vi "begin_DriveQuadTalonSrxl.vi"(0 "Time":T1, 3 "Gear Ratio":dbl=1.0 format="%.4f", 4 "Distance Type":T2, 5 "Enc Edges / Rev":dbl=1440.0 format="%.4f", 6 "Wheel Radius In":dbl=3.0 format="%.4f", 7 "MAX DESIRED\nVELOCITY\n(UNITS)":dbl=5800.0 format="%#_13g", 8 "Right Slave CAN":u8=12, 9 "RIght Master CAN":u8=10, 10 "Left Slave CAN":u8=13, 11 "Left Master CAN":u8=14) -> ()   [LabVIEW 2019, in "DriveQuadTalonSRX_Motor.lvlib"]
doc: "Open drives for 4 motor arcade drive using Talon SRX controllers. Configure for velocity control using directly wired encoders on master talon."
uses:
  DriveQuadTalonSRX_Motor.lvlib
  Dist_Type.ctl
  Time_Units_Control.ctl
  <vilib>/Rock Robotics/WPI/SafetyOutput/WPI_SafetyOutputConfigMenu.ctl
  <vilib>/Rock Robotics/WPI/ThirdParty/Phoenix-LabVIEW/Motor Controller/Controls/CTRE_Phoenix_MotorControl_FeedbackDevice.ctl
  <vilib>/Rock Robotics/WPI/ThirdParty/Phoenix-LabVIEW/Motor Controller/Controls/CTRE_Phoenix_MotorControl_NeutralMode.ctl
  globals_DriveQuadTalonSRX.vi
  <vilib>/Rock Robotics/WPI/RobotDrive/WPI_RobotDriveOpen2MotorWithExistingMotors.vi
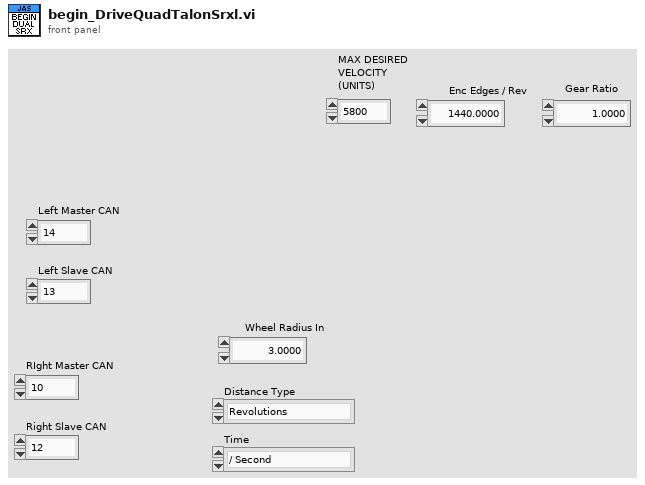
[diagram p1: front panel]
types:
  T1 = typedef "DriveQuadTalonSRX_Motor.lvlib/Time_Units_Control.ctl" = enum16{"/ Second", "/ Minute"}
  T2 = typedef "DriveQuadTalonSRX_Motor.lvlib/Dist_Type.ctl" = enum16{"Revolutions", "Feet"}
  T3 = typedef "CTRE_Phoenix_MotorControl_NeutralMode.ctl" = enum8{"EEPROMSetting", "Override to Coast", "Override to Brake"}
  T4 = typedef "WPI_SafetyOutputConfigMenu.ctl" = enum16{"Enable", "Disable"}
  T5 = enum16{"FollowerType_PercentOutput", "FollowerType_AuxOutput1"}
  T6 = typedef "CTRE_Phoenix_MotorControl_FeedbackDevice.ctl" = i8
  T7 = typedef "WPI_MotorControlDeviceRef.ctl" = cluster{"DeviceStatus":errorcluster, "Type":T8, "PWM":cluster{"PWM Channel":T9, "DeadBand":T10}, "CAN":cluster{"Device Number":u8, "SetOutput VI Ref":variant, "GetOutput VI Ref":variant, "Enable VI Ref":variant, "Disable VI Ref":variant, "Data":variant}, "Invert":bool, "DIO PWM":cluster{"PWM \"Enable\" Channel":T9, "DIOChannel":T11, "PWM Rate":dbl}}
  T8 = typedef "WPI_MotorControlType.ctl" = enum16{"PWM", "CAN", "DIO PWM"}
  T9 = typedef "FPGA_DIOPWMChannel.ctl" = enum8{"PWM 0", "PWM 1", "PWM 2", "PWM 3", "PWM 4", "PWM 5", "PWM 6", "PWM 7", "PWM 8", "PWM 9", "PWM MXP 0", "PWM MXP 1", "PWM MXP 2", "PWM MXP 3", "PWM MXP 4", "PWM MXP 5", "PWM MXP 6", "PWM MXP 7", "PWM MXP 8", "PWM MXP 9", "Invalid"}
  T10 = typedef "WPI_PWMDeadband.ctl" = cluster{"Name":string, "maxPositivePwm":i32, "minPositivePwm":i32, "centerPwm":i32, "maxNegativePwm":i32, "minNegativePwm":i32, "angularRange":u16}
  T11 = typedef "FPGA_DIOChannel.ctl" = enum8{"DIO 0", "DIO 1", "DIO 2", "DIO 3", "DIO 4", "DIO 5", "DIO 6", "DIO 7", "DIO 8", "DIO 9", "DIO MXP 0", "DIO MXP 1", "DIO MXP 2", "DIO MXP 3", "DIO MXP 4", "DIO MXP 5", "DIO MXP 6", "DIO MXP 7", "DIO MXP 8", "DIO MXP 9", "DIO MXP 10", "DIO MXP 11", "DIO MXP 12", "DIO MXP 13", "DIO MXP 14", "DIO MXP 15", "SPI Port CS1", "SPI Port CS2", "SPI Port CS3", "SPI Port MISO", "SPI Port MOSI", "Invalid"}
  T12 = typedef "WPI_RobotDriveDevRef.ctl" = cluster{"DevStatus":errorcluster, "Motors[]":T7[], "Square Inputs":bool, "Max Output":dbl}
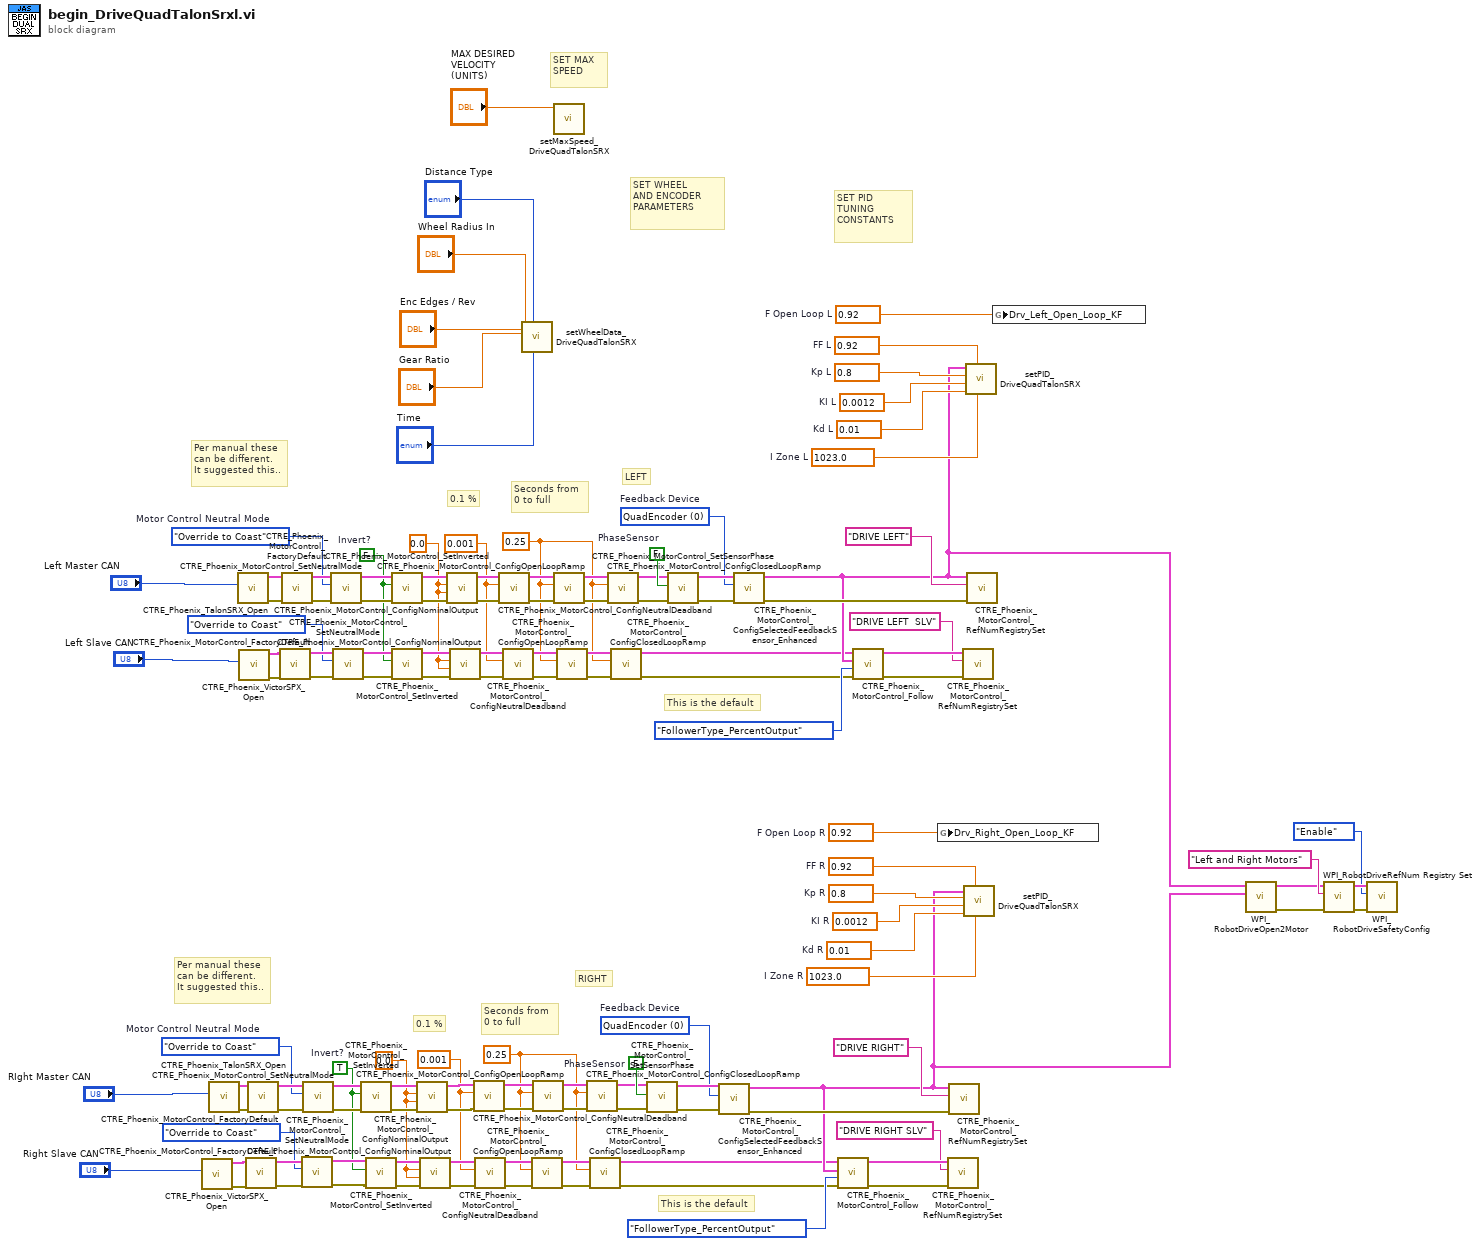
[diagram p0: block diagram]
diagram:
  w4 = 0.25 ("secondsFromNeutralToFull")
  w5 = 0.001 ("Percent Deadband")
  w6 = 0.0 ("Forward Nominal Percent Output")
  w27 = 0.25 ("secondsFromNeutralToFull")
  w28 = 0.001 ("Percent Deadband")
  w29 = 0.0 ("Forward Nominal Percent Output")
  w91 = 0.92  # F Open Loop L
  w97 = 1023.0  # I Zone L
  w98 = 0.01  # Kd L
  w99 = 0.0012  # KI L
  w100 = 0.8  # Kp L
  w101 = 0.92  # FF L
  w92 = 1023.0  # I Zone R
  w93 = 0.01  # Kd R
  w94 = 0.0012  # KI R
  w95 = 0.8  # Kp R
  w96 = 0.92  # FF R
  w90 = 0.92  # F Open Loop R
  w77 = FALSE  # Invert?
  w66 = TRUE  # Invert?
  w116 = T6 0 items=["None"=-1, "QuadEncoder"=0, "Analog"=2, "Tachometer"=4, "Pulse Width Encoded Position"=8, "Sensor Sum (S0 + S1)"=9, "Sensor Difference (D0 - D1)"=10, "Remote Source 0"=11, "Remote Source 1"=12, "Software Emulated"=15]  # Feedback Device
  w115 = T6 0 items=["None"=-1, "QuadEncoder"=0, "Analog"=2, "Tachometer"=4, "Pulse Width Encoded Position"=8, "Sensor Sum (S0 + S1)"=9, "Sensor Difference (D0 - D1)"=10, "Remote Source 0"=11, "Remote Source 1"=12, "Software Emulated"=15]  # Feedback Device
  w64 = CTRE_Phoenix_MotorControl_NeutralMode."Override to Coast"  # Motor Control Neutral Mode
  w76 = CTRE_Phoenix_MotorControl_NeutralMode."Override to Coast"  # Motor Control Neutral Mode
  w65 = FALSE  # PhaseSensor
  w104 = FALSE  # PhaseSensor
  # "This is the default"
  # "This is the default"
  # "Per manual these\ncan be different.  \nIt suggested this.."
  # "Per manual these\ncan be different.  \nIt suggested this.."
  # "Seconds from\n0 to full"
  # "Seconds from\n0 to full"
  # "0.1 %"
  # "0.1 %"
  # "SET PID\nTUNING\nCONSTANTS"
  # "SET WHEEL\nAND ENCODER\nPARAMETERS"
  # "SET MAX\nSPEED"
  # "RIGHT"
  # "LEFT"
  n1 = call <vilib>:"CTRE_Phoenix_VictorSPX_Open.vi"("Device Number"="Right Slave CAN") -> ("error out"=w63:errorcluster, "CAN Talon SRX Ref"=w62:T7)  [unwired: 9 in]
  n2 = call <vilib>:"CTRE_Phoenix_TalonSRX_Open.vi"("Device Number"="RIght Master CAN") -> ("error out"=w110:errorcluster, "CAN Talon SRX Ref"=w109:T7)  [unwired: 9 in]
  n3 = call <vilib>:"CTRE_Phoenix_TalonSRX_Open.vi"("Device Number"="Left Master CAN") -> ("error out"=w106:errorcluster, "CAN Talon SRX Ref"=w105:T7)  [unwired: 9 in]
  n4 = call <vilib>:"CTRE_Phoenix_VictorSPX_Open.vi"("Device Number"="Left Slave CAN") -> ("error out"=w60:errorcluster, "CAN Talon SRX Ref"=w59:T7)  [unwired: 9 in]
  n5 = call <vilib>:"CTRE_Phoenix_MotorControl_FactoryDefault.vi"("error in"=w63, "PhoenixMotorControlDevRef"=w62) -> ("error out"=w69:errorcluster, "PhoenixMotorControlDevRef"=w70:T7)  [unwired: 8 in]
  n6 = call <vilib>:"CTRE_Phoenix_MotorControl_FactoryDefault.vi"("error in"=w110, "PhoenixMotorControlDevRef"=w109) -> ("error out"=w114:errorcluster, "PhoenixMotorControlDevRef"=w113:T7)  [unwired: 8 in]
  n7 = call <vilib>:"CTRE_Phoenix_MotorControl_FactoryDefault.vi"("error in"=w60, "PhoenixMotorControlDevRef"=w59) -> ("error out"=w81:errorcluster, "PhoenixMotorControlDevRef"=w80:T7)  [unwired: 8 in]
  n8 = call <vilib>:"CTRE_Phoenix_MotorControl_FactoryDefault.vi"("error in"=w106, "PhoenixMotorControlDevRef"=w105) -> ("error out"=w112:errorcluster, "PhoenixMotorControlDevRef"=w111:T7)  [unwired: 8 in]
  n9 = call <vilib>:"CTRE_Phoenix_MotorControl_SetNeutralMode.vi"("error in (no error)"=w69, "Motor Control Neutral Mode"=CTRE_Phoenix_MotorControl_NeutralMode."Override to Coast", "PhoenixMotorControlDevRef"=w70) -> ("error out"=w75:errorcluster, "PhoenixMotorControlDevRef"=w74:T7)  [unwired: 7 in]
  n10 = call <vilib>:"CTRE_Phoenix_MotorControl_SetNeutralMode.vi"("error in (no error)"=w114, "Motor Control Neutral Mode"=w64, "PhoenixMotorControlDevRef"=w113) -> ("error out"=w121:errorcluster, "PhoenixMotorControlDevRef"=w122:T7)  [unwired: 7 in]
  n11 = call <vilib>:"CTRE_Phoenix_MotorControl_SetNeutralMode.vi"("error in (no error)"=w112, "Motor Control Neutral Mode"=w76, "PhoenixMotorControlDevRef"=w111) -> ("error out"=w118:errorcluster, "PhoenixMotorControlDevRef"=w117:T7)  [unwired: 7 in]
  n12 = call <vilib>:"CTRE_Phoenix_MotorControl_SetNeutralMode.vi"("error in (no error)"=w81, "Motor Control Neutral Mode"=CTRE_Phoenix_MotorControl_NeutralMode."Override to Coast", "PhoenixMotorControlDevRef"=w80) -> ("error out"=w78:errorcluster, "PhoenixMotorControlDevRef"=w79:T7)  [unwired: 7 in]
  n13 = call <vilib>:"CTRE_Phoenix_MotorControl_SetInverted.vi"("error in (no error)"=w121, "Invert?"=w66, "PhoenixMotorControlDevRef"=w122) -> ("error out"=w16:errorcluster, "PhoenixMotorControlDevRef"=w26:T7)  [unwired: 7 in]
  n14 = call <vilib>:"CTRE_Phoenix_MotorControl_SetInverted.vi"("error in (no error)"=w75, "Invert?"=w66, "PhoenixMotorControlDevRef"=w74) -> ("error out"=w11:errorcluster, "PhoenixMotorControlDevRef"=w21:T7)  [unwired: 7 in]
  n15 = call <vilib>:"CTRE_Phoenix_MotorControl_SetInverted.vi"("error in (no error)"=w118, "Invert?"=w77, "PhoenixMotorControlDevRef"=w117) -> ("error out"=w48:errorcluster, "PhoenixMotorControlDevRef"=w49:T7)  [unwired: 7 in]
  n16 = call <vilib>:"CTRE_Phoenix_MotorControl_SetInverted.vi"("error in (no error)"=w78, "Invert?"=w77, "PhoenixMotorControlDevRef"=w79) -> ("error out"=w36:errorcluster, "PhoenixMotorControlDevRef"=w37:T7)  [unwired: 7 in]
  n17 = call <vilib>:"CTRE_Phoenix_MotorControl_ConfigNominalOutput.vi"("error in (no error)"=w16, "Reverse Nominal Percent Output"=w6, "Forward Nominal Percent Output"=w6, "PhoenixMotorControlDevRef"=w26) -> ("error out"=w15:errorcluster, "PhoenixMotorControlDevRef"=w25:T7)  [unwired: 6 in]
  n18 = call <vilib>:"CTRE_Phoenix_MotorControl_ConfigNominalOutput.vi"("error in (no error)"=w11, "Reverse Nominal Percent Output"=w6, "Forward Nominal Percent Output"=w6, "PhoenixMotorControlDevRef"=w21) -> ("error out"=w10:errorcluster, "PhoenixMotorControlDevRef"=w20:T7)  [unwired: 6 in]
  n19 = call <vilib>:"CTRE_Phoenix_MotorControl_ConfigNominalOutput.vi"("error in (no error)"=w48, "Reverse Nominal Percent Output"=w29, "Forward Nominal Percent Output"=w29, "PhoenixMotorControlDevRef"=w49) -> ("error out"=w46:errorcluster, "PhoenixMotorControlDevRef"=w47:T7)  [unwired: 6 in]
  n20 = call <vilib>:"CTRE_Phoenix_MotorControl_ConfigNominalOutput.vi"("error in (no error)"=w36, "Reverse Nominal Percent Output"=w29, "Forward Nominal Percent Output"=w29, "PhoenixMotorControlDevRef"=w37) -> ("error out"=w32:errorcluster, "PhoenixMotorControlDevRef"=w35:T7)  [unwired: 6 in]
  n21 = call <vilib>:"CTRE_Phoenix_MotorControl_ConfigNeutralDeadband.vi"("error in (no error)"=w15, "Percent Deadband"=w5, "PhoenixMotorControlDevRef"=w25) -> ("error out"=w14:errorcluster, "PhoenixMotorControlDevRef"=w24:T7)  [unwired: 7 in]
  n22 = call <vilib>:"CTRE_Phoenix_MotorControl_ConfigNeutralDeadband.vi"("error in (no error)"=w10, "Percent Deadband"=w5, "PhoenixMotorControlDevRef"=w20) -> ("error out"=w9:errorcluster, "PhoenixMotorControlDevRef"=w19:T7)  [unwired: 7 in]
  n23 = call <vilib>:"CTRE_Phoenix_MotorControl_ConfigNeutralDeadband.vi"("error in (no error)"=w46, "Percent Deadband"=w28, "PhoenixMotorControlDevRef"=w47) -> ("error out"=w44:errorcluster, "PhoenixMotorControlDevRef"=w45:T7)  [unwired: 7 in]
  n24 = call <vilib>:"CTRE_Phoenix_MotorControl_ConfigNeutralDeadband.vi"("error in (no error)"=w32, "Percent Deadband"=w28, "PhoenixMotorControlDevRef"=w35) -> ("error out"=w31:errorcluster, "PhoenixMotorControlDevRef"=w34:T7)  [unwired: 7 in]
  n25 = call "setWheelData_DriveQuadTalonSRX.vi"("Time"="Time", "Distance Type"="Distance Type", "Enc Edges / Rev"="Enc Edges / Rev", "Gear Ratio"="Gear Ratio", "Wheel Radius In"="Wheel Radius In") -> ()  [unwired: 2 in, 5 out]
  n26 = call <vilib>:"CTRE_Phoenix_MotorControl_ConfigOpenLoopRamp.vi"("error in (no error)"=w9, "secondsFromNeutralToFull"=w4, "PhoenixMotorControlDevRef"=w19) -> ("error out"=w8:errorcluster, "PhoenixMotorControlDevRef"=w18:T7)  [unwired: 7 in]
  n27 = call <vilib>:"CTRE_Phoenix_MotorControl_ConfigOpenLoopRamp.vi"("error in (no error)"=w14, "secondsFromNeutralToFull"=w4, "PhoenixMotorControlDevRef"=w24) -> ("error out"=w13:errorcluster, "PhoenixMotorControlDevRef"=w23:T7)  [unwired: 7 in]
  n28 = call "setMaxSpeed_DriveQuadTalonSRX.vi"("MAX DESIRED\nVELOCITY (UNITS)"="MAX DESIRED\nVELOCITY\n(UNITS)") -> ()  [unwired: 8 in, 2 out]
  n29 = call <vilib>:"CTRE_Phoenix_MotorControl_ConfigOpenLoopRamp.vi"("error in (no error)"=w44, "secondsFromNeutralToFull"=w27, "PhoenixMotorControlDevRef"=w45) -> ("error out"=w42:errorcluster, "PhoenixMotorControlDevRef"=w43:T7)  [unwired: 7 in]
  n30 = call <vilib>:"CTRE_Phoenix_MotorControl_ConfigOpenLoopRamp.vi"("error in (no error)"=w31, "secondsFromNeutralToFull"=w27, "PhoenixMotorControlDevRef"=w34) -> ("error out"=w30:errorcluster, "PhoenixMotorControlDevRef"=w33:T7)  [unwired: 7 in]
  n31 = call <vilib>:"CTRE_Phoenix_MotorControl_ConfigClosedLoopRamp.vi"("error in (no error)"=w13, "secondsFromNeutralToFull"=w4, "PhoenixMotorControlDevRef"=w23) -> ("error out"=w12:errorcluster, "PhoenixMotorControlDevRef"=w22:T7)  [unwired: 7 in]
  n32 = call <vilib>:"CTRE_Phoenix_MotorControl_ConfigClosedLoopRamp.vi"("error in (no error)"=w8, "secondsFromNeutralToFull"=w4, "PhoenixMotorControlDevRef"=w18) -> ("error out"=w7:errorcluster, "PhoenixMotorControlDevRef"=w17:T7)  [unwired: 7 in]
  n33 = call <vilib>:"CTRE_Phoenix_MotorControl_ConfigClosedLoopRamp.vi"("error in (no error)"=w42, "secondsFromNeutralToFull"=w27, "PhoenixMotorControlDevRef"=w43) -> ("error out"=w41:errorcluster, "PhoenixMotorControlDevRef"=w40:T7)  [unwired: 7 in]
  n34 = call <vilib>:"CTRE_Phoenix_MotorControl_ConfigClosedLoopRamp.vi"("error in (no error)"=w30, "secondsFromNeutralToFull"=w27, "PhoenixMotorControlDevRef"=w33) -> ("error out"=w39:errorcluster, "PhoenixMotorControlDevRef"=w38:T7)  [unwired: 7 in]
  n35 = call <vilib>:"CTRE_Phoenix_MotorControl_SetSensorPhase.vi"("error in (no error)"=w12, "PhaseSensor"=w65, "PhoenixMotorControlDevRef"=w22) -> ("error out"=w123:errorcluster, "PhoenixMotorControlDevRef"=w124:T7)  [unwired: 7 in]
  n36 = call <vilib>:"CTRE_Phoenix_MotorControl_SetSensorPhase.vi"("error in (no error)"=w41, "PhaseSensor"=w104, "PhoenixMotorControlDevRef"=w40) -> ("error out"=w120:errorcluster, "PhoenixMotorControlDevRef"=w119:T7)  [unwired: 7 in]
  n37 = call <vilib>:"CTRE_Phoenix_MotorControl_ConfigSelectedFeedbackSensor_Enhanced.vi"("error in (no error)"=w123, "Feedback Device"=w115, "PhoenixMotorControlDevRef"=w124) -> ("error out"=w125:errorcluster, "PhoenixMotorControlDevRef"=w50:T7)  [unwired: 7 in]
  n38 = call <vilib>:"CTRE_Phoenix_MotorControl_ConfigSelectedFeedbackSensor_Enhanced.vi"("error in (no error)"=w120, "Feedback Device"=w116, "PhoenixMotorControlDevRef"=w119) -> ("error out"=w126:errorcluster, "PhoenixMotorControlDevRef"=w51:T7)  [unwired: 7 in]
  n39 = call <vilib>:"CTRE_Phoenix_MotorControl_Follow.vi"("error in (no error)"=w7, "FollowerType"=T5."FollowerType_PercentOutput", "Master Controller to Follow"=w50, "PhoenixMotorControlDevRef"=w17) -> ("error out"=w73:errorcluster, "PhoenixMotorControlDevRef"=w72:T7)  [unwired: 6 in]
  n40 = call <vilib>:"CTRE_Phoenix_MotorControl_Follow.vi"("error in (no error)"=w39, "FollowerType"=T5."FollowerType_PercentOutput", "Master Controller to Follow"=w51, "PhoenixMotorControlDevRef"=w38) -> ("error out"=w84:errorcluster, "PhoenixMotorControlDevRef"=w83:T7)  [unwired: 6 in]
  n41 = global write "globals_DriveQuadTalonSRX.vi" "Drv_Right_Open_Loop_KF"(w90) -> ()
  n42 = call <vilib>:"CTRE_Phoenix_MotorControl_RefNumRegistrySet.vi"("error in (no error)"=w73, "refnum name"="DRIVE RIGHT SLV", "PhoenixMotorControlDevRef"=w72) -> ()  [unwired: 7 in, 2 out]
  n43 = call <vilib>:"CTRE_Phoenix_MotorControl_RefNumRegistrySet.vi"("error in (no error)"=w125, "refnum name"="DRIVE RIGHT", "PhoenixMotorControlDevRef"=w50) -> ()  [unwired: 7 in, 2 out]
  n44 = call <vilib>:"CTRE_Phoenix_MotorControl_RefNumRegistrySet.vi"("error in (no error)"=w84, "refnum name"="DRIVE LEFT  SLV", "PhoenixMotorControlDevRef"=w83) -> ()  [unwired: 7 in, 2 out]
  n45 = call "setPID_DriveQuadTalonSRX.vi"("I ZONE"=w92, "FF"=w96, "KD"=w93, "KI"=w94, "KP"=w95, "MasterDriveRef"=w50) -> ()  [unwired: 6 in]
  n46 = call "setPID_DriveQuadTalonSRX.vi"("I ZONE"=w97, "FF"=w101, "KD"=w98, "KI"=w99, "KP"=w100, "MasterDriveRef"=w51) -> ()  [unwired: 6 in]
  n47 = call <vilib>:"CTRE_Phoenix_MotorControl_RefNumRegistrySet.vi"("error in (no error)"=w126, "refnum name"="DRIVE LEFT", "PhoenixMotorControlDevRef"=w51) -> ()  [unwired: 7 in, 2 out]
  n48 = global write "globals_DriveQuadTalonSRX.vi" "Drv_Left_Open_Loop_KF"(w91) -> ()
  n49 = call-poly <vilib>:"WPI_RobotDriveOpen2Motor.vi"("Right Motor Dev Ref"=w50, "Left Motor Dev Ref"=w51) -> ("error out"=w54:errorcluster, "RobotDriveDevRef"=w52:T12)  [unwired: 8 in]
  n50 = call <vilib>:"WPI_RobotDriveRefNum Registry Set.vi"("error in (no error)"=w54, "refnum name"="Left and Right Motors", "RobotDriveDevRef"=w52) -> ("error out"=w57:errorcluster, "RobotDriveDevRef"=w56:T12)  [unwired: 7 in]
  n51 = call <vilib>:"WPI_RobotDriveSafetyConfig.vi"("error in (no error)"=w57, "mode"=WPI_SafetyOutputConfigMenu."Enable", "RobotDriveDevRef"=w56) -> ()  [unwired: 7 in, 2 out]
